vi "FPGAPowerMeasurement2.vi"() -> ()   [LabVIEW 2009]
panel:
  out "Average Power":dbl
  out "Average Voltage":dbl
  out "Average Current":dbl
  out "Power":dynamicdata(graph)
  out "Current":dynamicdata(graph)
  out "Voltage at FPGA":dynamicdata(graph)
  in  "stop":bool
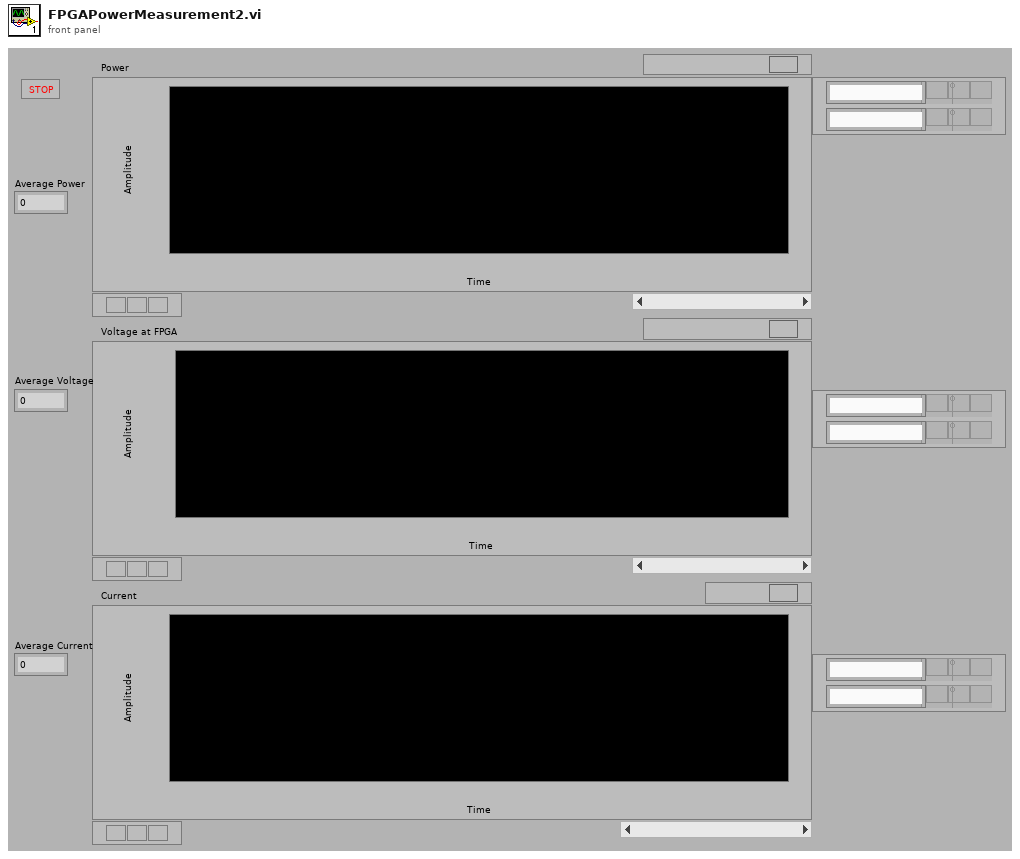
[diagram p1: front panel]
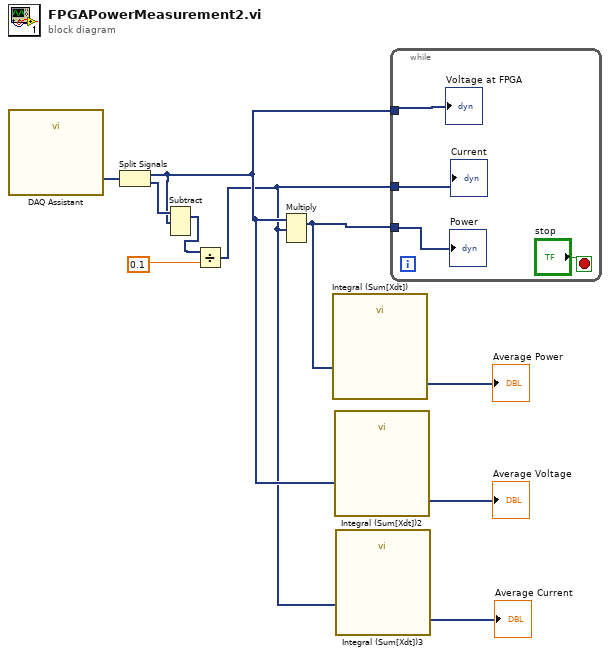
[diagram p0: block diagram]
diagram:
  n1 = call "DAQ Assistant"() -> ("data"=w6:dynamicdata)  [unwired: 17 in, 2 out]
  n2 = Split Signals(w6) -> (w4:dynamicdata, w5:dynamicdata)  [unwired: 2 in]
  n3 = Subtract(1:w4, 2:w5) -> (0:w3:dynamicdata)  [unwired: 1 in, 1 out]
  n4 = Divide(x=w3, y=0.1) -> (x/y=w2:dynamicdata)
  n5 = Multiply(1:w2, 2:w4) -> (0:w10:dynamicdata)  [unwired: 1 in, 1 out]
  n6 = call "Integral (Sum[Xdt])"("Signals"=w10) -> ("Result"=→"Average Power":dynamicdata)  [unwired: 5 in, 1 out]
  n7 = call "Integral (Sum[Xdt])2"("Signals"=w4) -> ("Result"=→"Average Voltage":dynamicdata)  [unwired: 5 in, 1 out]
  n8 = call "Integral (Sum[Xdt])3"("Signals"=w2) -> ("Result"=→"Average Current":dynamicdata)  [unwired: 5 in, 1 out]
  n9 = while {
    tunnel: w4 -> [w13]
    tunnel: w2 -> [w12]
    tunnel: w10 -> [w11]
    stop <- "stop" stop-if-true
    "Voltage at FPGA" <- w13
    "Current" <- w12
    "Power" <- w11
  }
